vi "Actuate HW.vi"(8 "error in (no error)":errorcluster, 11 "Simulated Switch in":refnum<class "Simulated Switch.lvclass">) -> (0 "error out":errorcluster, 3 "Simulated Switch out":refnum<class "Simulated Switch.lvclass">)   [LabVIEW 2020, in "Simulated Switch.lvclass"]
uses:
  Simulated Switch.lvclass
  C:/Users/jharw/Documents/1 Folder to Rule them All/UMD/Inflation-Apparatus/src/Hardware/General Hardware.lvclass
  C:/Users/jharw/Documents/1 Folder to Rule them All/UMD/Inflation-Apparatus/src/Hardware/Actuators/Switches/Switch.lvclass
  General Hardware.lvclass/General Hardware.ctl
  Switch.lvclass/Switch.ctl
  Switch.lvclass
  General Hardware.lvclass
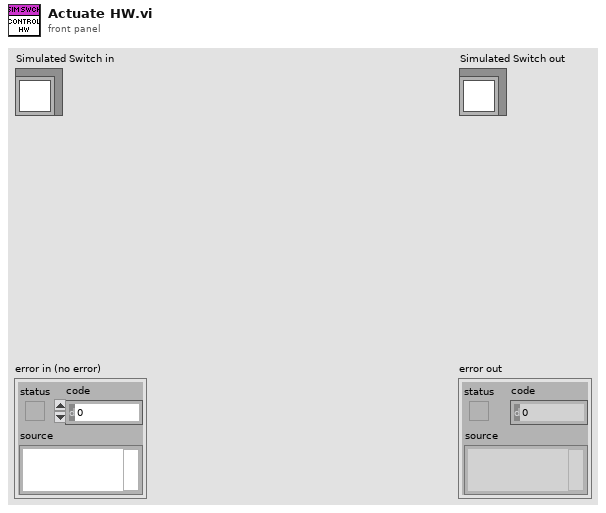
[diagram p1: front panel]
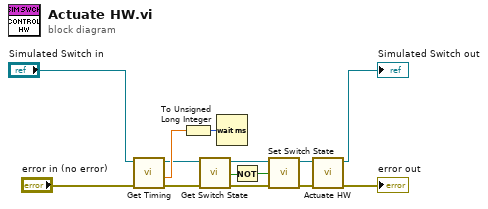
[diagram p0: block diagram]
diagram:
  n1 = call "Get Timing.vi"("error in (no error)"="error in (no error)", "General Hardware in"="Simulated Switch in") -> ("error out"=w9:errorcluster, "time delay (ms)"=w12:dbl, "General Hardware out"=w10:refnum<class "Simulated Switch.lvclass">)  [unwired: 6 in, 1 out]
  n2 = To Unsigned Long Integer(number=w12) -> (unsigned 32bit integer=w11:u32)
  n3 = call "Get Switch State.vi"("error in (no error)"=w9, "Switch in"=w10) -> ("error out"=w5:errorcluster, "switch state"=w8:bool, "Switch out"=w7:refnum<class "Simulated Switch.lvclass">)  [unwired: 7 in]
  n4 = Wait (ms)(milliseconds to wait=w11) -> ()  [unwired: 1 out]
  n5 = Not(x=w8) -> (.not. x?=w6:bool)
  n6 = call "Set Switch State.vi"("error in (no error)"=w5, "switch state"=w6, "Switch in"=w7) -> ("error out"=w2:errorcluster, "Switch out"=w4:refnum<class "Simulated Switch.lvclass">)  [unwired: 7 in]
  n7 = call-parent "Actuate HW.vi"("error in (no error)"=w2, "Switch in"=w4) -> ("error out"=→"error out":errorcluster, "Switch out"=→"Simulated Switch out":refnum<class "Simulated Switch.lvclass">)  [unwired: 8 in]
